vi "Configure Trigger A Direction.vi"(8 "error in (no error)":errorcluster, 9 "Direction (In)":i32(ring) items=["In", "Out"], 10 "Trigger (1)":i32=1, 11 "VISA resource name":refnum<visa-resource-name>) -> (0 "error out":errorcluster, 3 "VISA resource name out":refnum<visa-resource-name>)   [LabVIEW 2015, in "Rohde&Schwarz CMXP Base.lvlib"]
doc: "Configures the trigger connectors of an R&SCMW as input or output connectors.\n\nAttributes:\nRSCMXPBASE_ATTR_SELECT_TRIGGER\nRSCMXPBASE_ATTR_TRIGGER_A_DIRECTION\n\nRemote-control command:\nTRIGger:BASE:EXTA<n>:DIRection"
uses:
  <instrlib>/Rohde&Schwarz CMXP Base/Rohde&Schwarz CMXP Base.lvlib
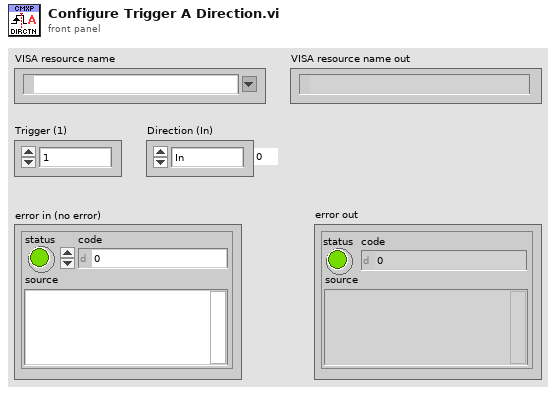
[diagram p1: front panel]
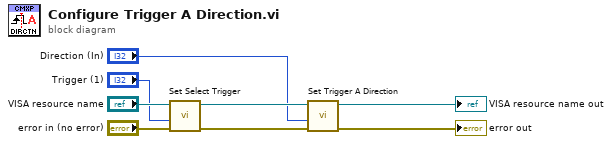
[diagram p0: block diagram]
diagram:
  n1 = call "Set Select Trigger"("error in (no error)"="error in (no error)", "Select Trigger (0)"="Trigger (1)", "instrument handle"="VISA resource name") -> ("error out"=w3:errorcluster, "instrument handle out"=w4:refnum<visa-resource-name>)  [unwired: 7 in]
  n2 = call "Set Trigger A Direction"("error in (no error)"=w3, "Trigger A Direction (0 - In)"="Direction (In)", "instrument handle"=w4) -> ("error out"=→"error out":errorcluster, "instrument handle out"=→"VISA resource name out":refnum<visa-resource-name>)  [unwired: 7 in]
